vi "CheckIfGObjectMatches.vi"(8 "error in (no error)":errorcluster, 10 "GObj Refnum":refnum<vi>, 11 "Ring Layout in":refnum<class "Ring Layout.lvclass">) -> (0 "error out":errorcluster, 2 "compatible?":bool)   [LabVIEW 2010, in "NI_SE_Front Panel Layout.lvlib" / "Ring Layout.lvclass"]
uses:
  Ring Layout.lvclass
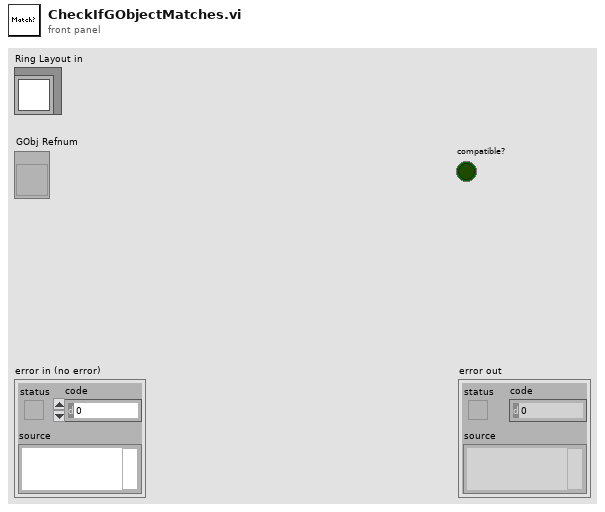
[diagram p1: front panel]
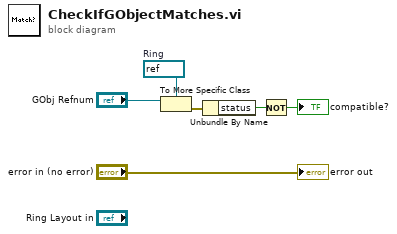
[diagram p0: block diagram]
diagram:
  w6 = refnum<vi> refnum  # Ring
  n1 = To More Specific Class(target class=w6, reference="GObj Refnum") -> (error out=w5:errorcluster)  [unwired: 1 in, 1 out]
  n2 = Unbundle By Name(w5) -> ("status"=w4:bool)
  n3 = Not(x=w4) -> (.not. x?=→"compatible?":bool)
  "error out" <- "error in (no error)"
